vi "Telnet_Send.vi"(8 "Error In":errorcluster caption="Entrée d'erreur", 10 "Data in":string, 11 "telnet connection in":T1) -> (0 "Error Out":errorcluster caption="Sortie d'erreur", 3 "telnet connection out":T1)   [LabVIEW 2013]
uses:
  <vilib>/addons/internet/telnet/telnet.llb/Telnet Session.ctl
  <vilib>/addons/internet/NI_InternetTK_Core_VIs.lvlib
panel:
  out "bytes written":i32
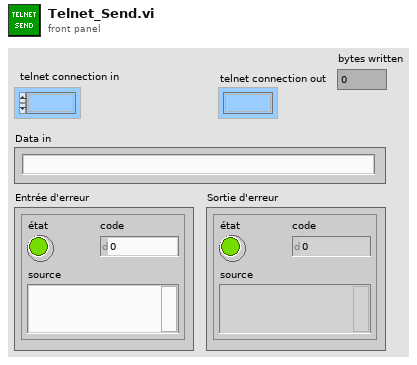
[diagram p1: front panel]
types:
  T1 = typedef "Telnet Session.ctl" = refnum<k1>
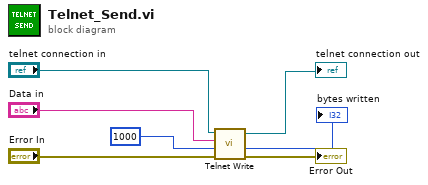
[diagram p0: block diagram]
diagram:
  n1 = call <vilib>:"Telnet Write.vi"("error in (no error)"="Error In", "timeout ms (25000)"=1000, "data in"="Data in", "telnet connection"="telnet connection in") -> ("error out"=→"Error Out":errorcluster, "bytes written"=→"bytes written":i32, "telnet connection out"=→"telnet connection out":T1)  [unwired: 3 in]
